vi "Self Test.vi"(8 "error in":errorcluster, 10 "Board Image":T1, 11 "FPGA in":refnum<class "FPGA Chip.lvclass">) -> (0 "error out":errorcluster, 2 "Pass?":T2, 3 "FPGA out":refnum<class "FPGA Chip.lvclass">)   [LabVIEW 2023, in "FPGA Chip.lvclass"]
doc: "Check the image for this component's placement on the board."
uses:
  FPGA Chip.lvclass
  Common/Pass Fail Boolean.ctl
  c:/dev/_r/4/eng/lv-core/lvpostprocessingd/lv_mc_x86_64/dist_i386/examples/Object-Oriented Programming/Board Testing/Object Design/Component/Component.lvclass
  Common/Board Image.ctl
  Component/Component.lvclass
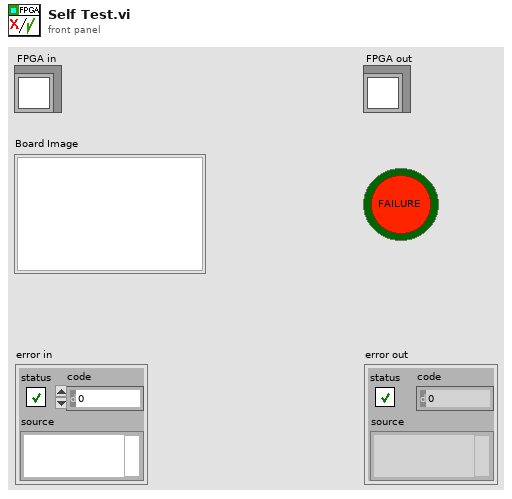
[diagram p1: front panel]
types:
  T1 = typedef "Board Image.ctl" = picture
  T2 = typedef "Pass Fail Boolean.ctl" = bool
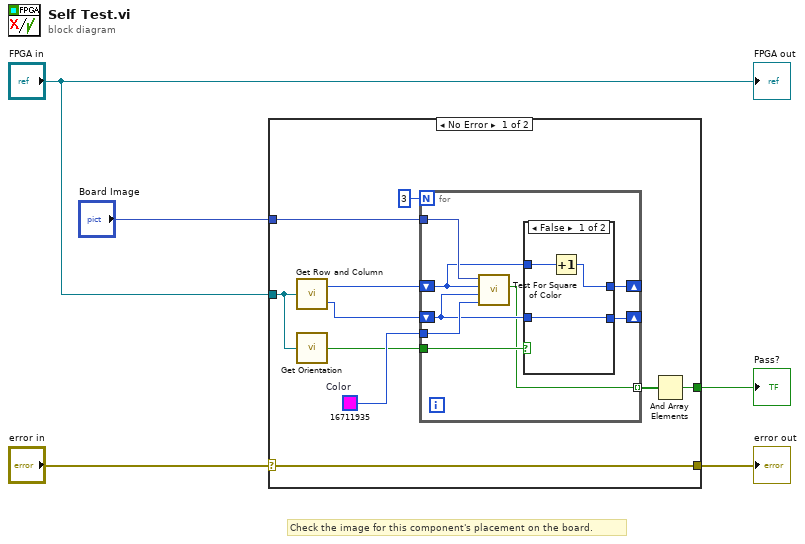
[diagram p0: block diagram]
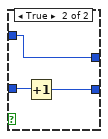
[diagram p2: hidden frame]
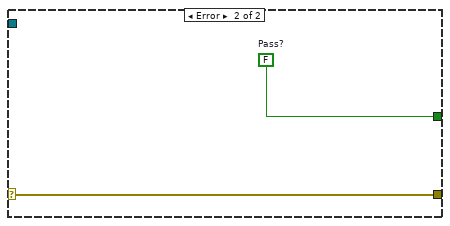
[diagram p3: hidden frame]
diagram:
  # "Check the image for this component's placement on the board."
  n1 = case shown="No Error" "error in" {
    selector: "error in" -> [w15 w31]
    tunnel: [w15 w31] -> w4
    tunnel: [w12 w30] -> w3
    tunnel: "FPGA in" -> [w10 _]
    tunnel: "Board Image" -> [w6 _]
    frame No Error {
      w11 = u32 16711935  # Color
      n2 = call "Get Row and Column.vi"("Component in"=w10) -> ("row"=w9:i16, "column"=w8:i16)
      n3 = call "Get Orientation.vi"("Component.lvclass"=w10) -> ("landscape?"=w7:bool)
      n4 = for {
        N: 3 -> [_]
        tunnel: w11 -> [w23]
        tunnel: w6 -> [w22]
        shift-right: [w17] -> _
        shift-left: w9 -> [w19]
        shift-right: [w18] -> _
        shift-left: w8 -> [w20]
        tunnel: w7 -> [w21]
        tunnel: [w16] -> w13 mode=indexing
        n5 = call "Test For Square of Color.vi"("color"=w23, "column"=w20, "row"=w19, "board image"=w22) -> ("pass?"=w16:T2)  [unwired: 7 in]
        n6 = case shown="False" w21 {
          tunnel: w20 -> [w24 w29]
          tunnel: w19 -> [w26 w27]
          tunnel: [w24 w28] -> w18
          tunnel: [w25 w27] -> w17
          frame False {
            n7 = Increment(x=w26) -> (x+1=w25:i16)
          }
          frame True {
            n8 = Increment(x=w29) -> (x+1=w28:i16)
          }
        }
      }
      n9 = And Array Elements(Boolean array=w13) -> (logical AND=w12:bool)
    }
    frame Error {
      w30 = T2 FALSE  # Pass?
    }
  }
  "error out" <- w4
  "Pass?" <- w3
  "FPGA out" <- "FPGA in"
